vi "Absorbance.vi"(10 "Longueur d'onde":dbl) -> (2 "absorbance":dbl)   [LabVIEW 2022 SP3]
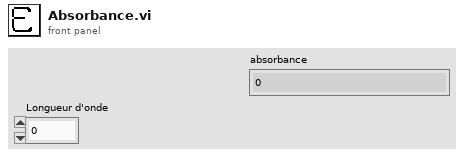
[diagram p1: front panel]
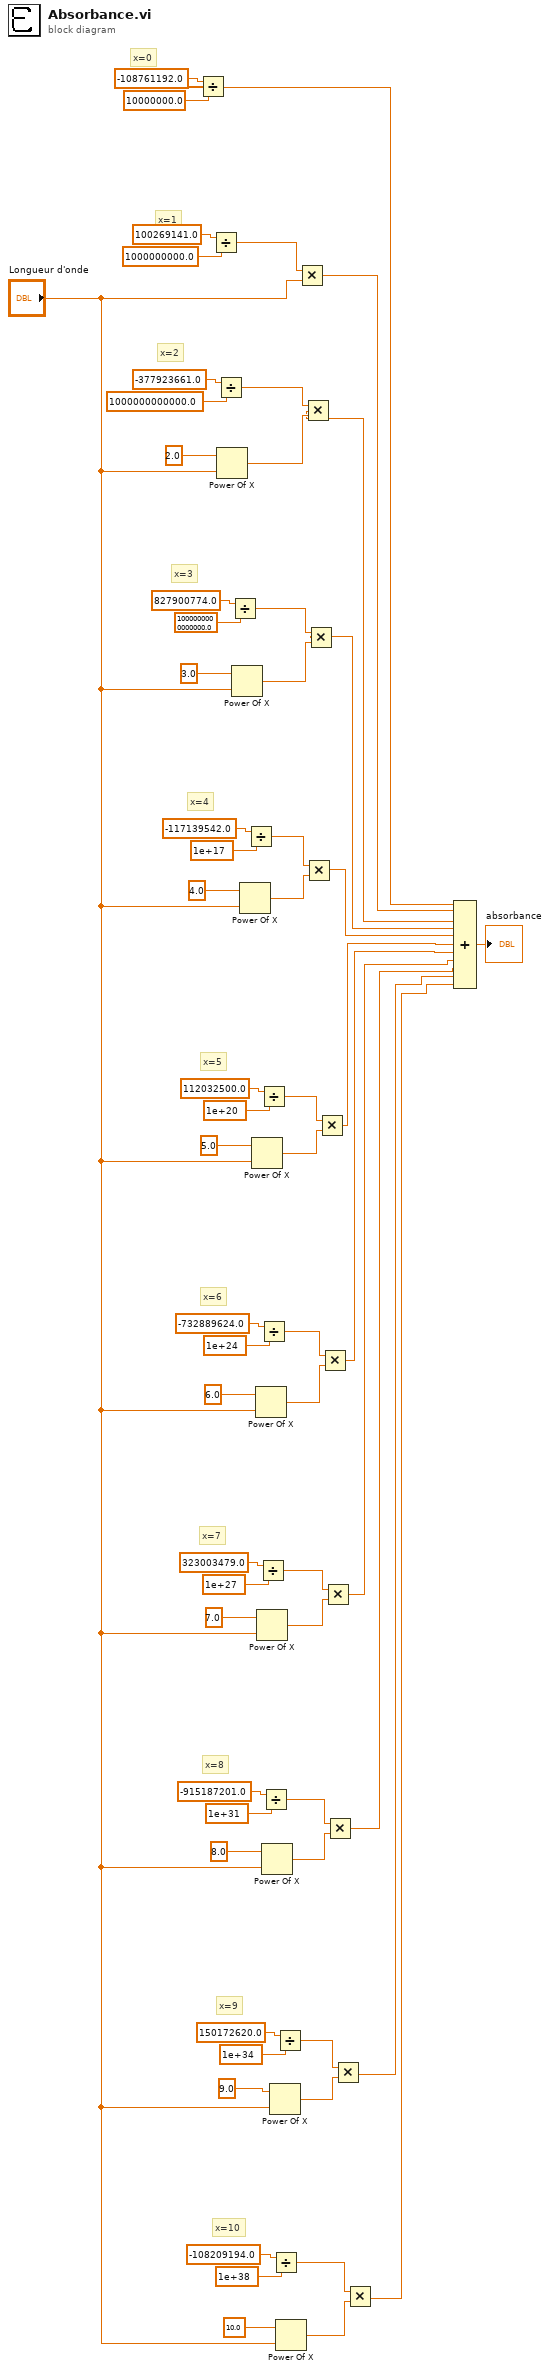
[diagram p0: block diagram]
diagram:
  # "x=10"
  # "x=9"
  # "x=8"
  # "x=7"
  # "x=6"
  # "x=5"
  # "x=4"
  # "x=3"
  # "x=2"
  # "x=1"
  # "x=0"
  n1 = Divide(x=-108761192.0, y=10000000.0) -> (x/y=w12:dbl)
  n2 = Divide(x=100269141.0, y=1000000000.0) -> (x/y=w32:dbl)
  n3 = Divide(x=-377923661.0, y=1000000000000.0) -> (x/y=w31:dbl)
  n4 = Power Of X(1:"Longueur d'onde", 2:2.0 ("y")) -> (0:w30:dbl)
  n5 = Divide(x=827900774.0, y=1000000000000000.0) -> (x/y=w28:dbl)
  n6 = Power Of X(1:"Longueur d'onde", 2:3.0 ("y")) -> (0:w27:dbl)
  n7 = Power Of X(1:"Longueur d'onde", 2:4.0 ("y")) -> (0:w25:dbl)
  n8 = Divide(x=-117139542.0, y=1e+17) -> (x/y=w26:dbl)
  n9 = Power Of X(1:"Longueur d'onde", 2:5.0 ("y")) -> (0:w23:dbl)
  n10 = Power Of X(1:"Longueur d'onde", 2:6.0 ("y")) -> (0:w21:dbl)
  n11 = Power Of X(1:"Longueur d'onde", 2:7.0 ("y")) -> (0:w19:dbl)
  n12 = Divide(x=323003479.0, y=1e+27) -> (x/y=w20:dbl)
  n13 = Divide(x=112032500.0, y=1e+20) -> (x/y=w24:dbl)
  n14 = Divide(x=-732889624.0, y=1e+24) -> (x/y=w22:dbl)
  n15 = Divide(x=-915187201.0, y=1e+31) -> (x/y=w18:dbl)
  n16 = Power Of X(1:"Longueur d'onde", 2:8.0 ("y")) -> (0:w17:dbl)
  n17 = Power Of X(1:"Longueur d'onde", 2:9.0 ("y")) -> (0:w15:dbl)
  n18 = Divide(x=-108209194.0, y=1e+38) -> (x/y=w14:dbl)
  n19 = Divide(x=150172620.0, y=1e+34) -> (x/y=w16:dbl)
  n20 = Power Of X(1:"Longueur d'onde", 2:10.0 ("y")) -> (0:w13:dbl)
  n21 = Multiply(x=w32, y="Longueur d'onde") -> (x*y=w11:dbl)
  n22 = Multiply(x=w31, y=w30) -> (x*y=w10:dbl)
  n23 = Multiply(x=w26, y=w25) -> (x*y=w8:dbl)
  n24 = Multiply(x=w28, y=w27) -> (x*y=w9:dbl)
  n25 = Multiply(x=w24, y=w23) -> (x*y=w7:dbl)
  n26 = Multiply(x=w22, y=w21) -> (x*y=w6:dbl)
  n27 = Multiply(x=w20, y=w19) -> (x*y=w5:dbl)
  n28 = Multiply(x=w18, y=w17) -> (x*y=w4:dbl)
  n29 = Multiply(x=w16, y=w15) -> (x*y=w3:dbl)
  n30 = Multiply(x=w14, y=w13) -> (x*y=w2:dbl)
  n31 = Compound Arithmetic op=ADD(w12, w11, w10, w9, w8, w7, w6, w5, w4, w3, w2) -> (→"absorbance":dbl)
